vi "Temperature.vi"() -> (3 "Array":dbl[](array[numeric]))   [LabVIEW 2019]
uses:
  <vilib>/numeric/Random Number (Range) DBL.vi
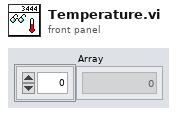
[diagram p1: front panel]
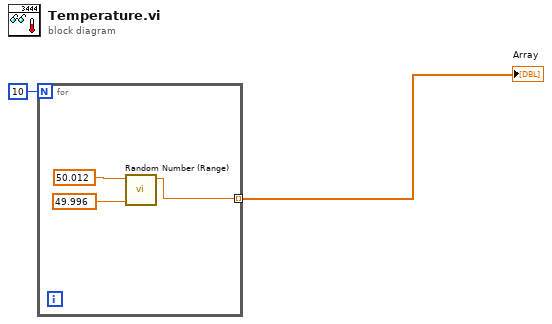
[diagram p0: block diagram]
diagram:
  n1 = for {
    N: 10 -> [_]
    tunnel: [w3] -> w1 mode=indexing
    n2 = call-poly <vilib>:"Random Number (Range).vi"("lower bound (0)"=49.996, "upper bound (100)"=50.012) -> ("number"=w3:dbl)  [unwired: 9 in]
  }
  "Array" <- w1
